vi "write to port.vi"(0 "number to write to port":i8) -> ()   [LabVIEW 2014]
uses:
  Instance           1 21Saved   write to port .vi
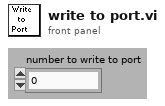
[diagram p1: front panel]
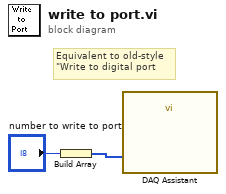
[diagram p0: block diagram]
diagram:
  # "Equivalent to old-style\n\"Write to digital port"
  n1 = Build Array("number to write to port") -> (w1:i8[])
  n2 = call "DAQ Assistant"("data"=w1) -> ()  [unwired: 9 in, 2 out]
